vi "GenerateCode.vi"(1 "Terms":T1[](array[typedef]), 3 "Diagram":refnum<vi>, 5 "XRef":refnum<vi>, 6 "State In":T4) -> (0 "Generated Code?":bool, 2 "State Out":T4, 4 "Reply":string[](array[string]))   [LabVIEW 2012, in "Unindex and Unbundle.xnode"]
doc: "This ability VI is called when it is time to define the execution behavior of your XNode via LabVIEW's scripting API. This VI is only called when you have previously informed LabVIEW that you need to script through a GenerateCode reply. Diagram is a reference to a diagram of a temporary VI. This diagram contains exactly one front panel terminal for each terminal of your XNode. Terms is an array of pairs of Term IDs and terminal references. LabVIEW will copy code scripted into this diagram into your XNode and connect everything to the correct terminals. The front panel terminals that are on this diagram are special in that they can only be on the top level diagram.\n \n Generate Code? is used to tell LabVIEW whether or not you want to copy the scripted diagram over. If there is an error and you wish not to commit the changes, then the old XNode behavior will be left unchanged. If you set Generate Code? to false, then this VI will be called again next time type propagation is run. Otherwise, it will not be called until you indicate that it should be through the reply on another ability VI.\n \n Because the diagram you are scripting into is separate from the VI containing the XNode instance, type propagation and the data manager will run on the temporary VI after each scripting call.\n \n You should not use the Copy scripting method to move code into the temporary VI. This will adversely affect the user's clipboard. You should use the Move scripting method instead.\n\nDefault behavior: None.\n\nThis ability does not provide UI and OS messages are not handled.\n\nSee also: ModifyCode"
uses:
  Unindex and Unbundle.xnode
  State.ctl
  <vilib>/XNodeSupport/XNodeTermIDPair.ctl
  <vilib>/XNodeSupport/XNodeTermRef.ctl
  <vilib>/XNodeSupport/XNodeString.ctl
  <vilib>/Utility/miscctls.llb/LVPositionTypeDef.ctl
  VI Scripting/Scripting Tools/Scripting Tools.lvlib
  <vilib>/XNodeSupport/NI_XNodeSupport.lvlib
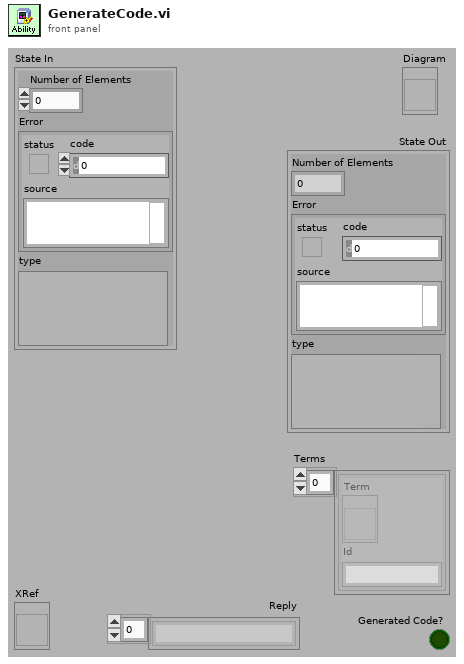
[diagram p1: front panel]
types:
  T1 = typedef "NI_XNodeSupport.lvlib/XNodeTermIDPair.ctl" = cluster{"Term":T2, "Id":T3}
  T2 = typedef "NI_XNodeSupport.lvlib/XNodeTermRef.ctl" = refnum<vi>
  T3 = typedef "NI_XNodeSupport.lvlib/XNodeString.ctl" = string
  T4 = typedef "Unindex and Unbundle.xnode/State.ctl" = cluster{"Number of Elements":i32, "Error":errorcluster, "type":variant}
  T5 = typedef "LVPositionTypeDef.ctl" = cluster{"Left":i32, "Top":i32}
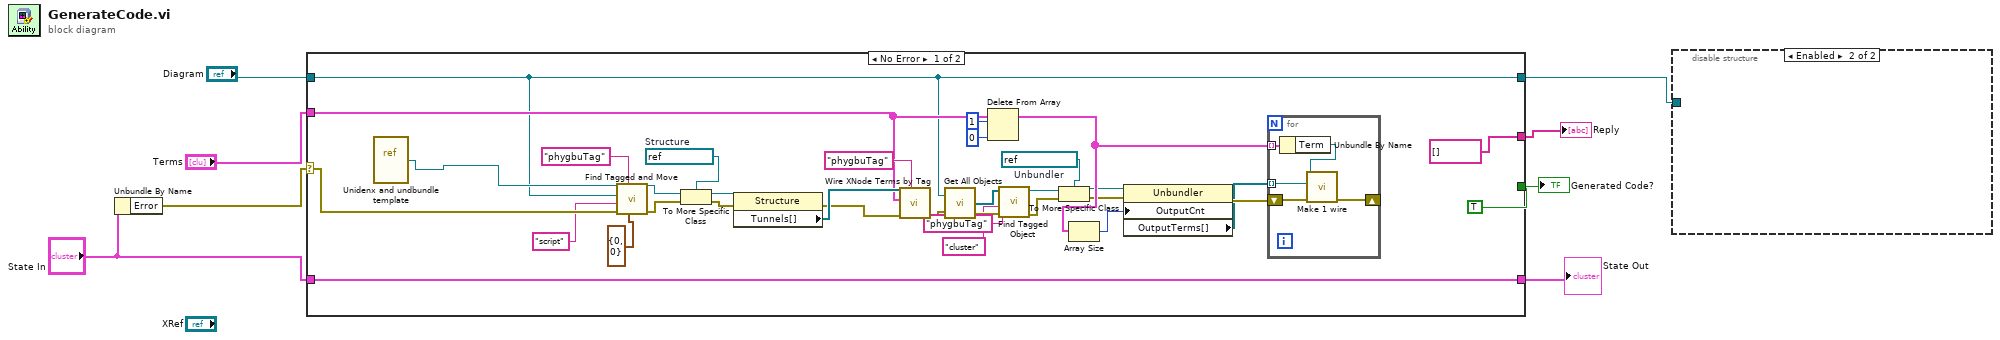
[diagram p0: block diagram]
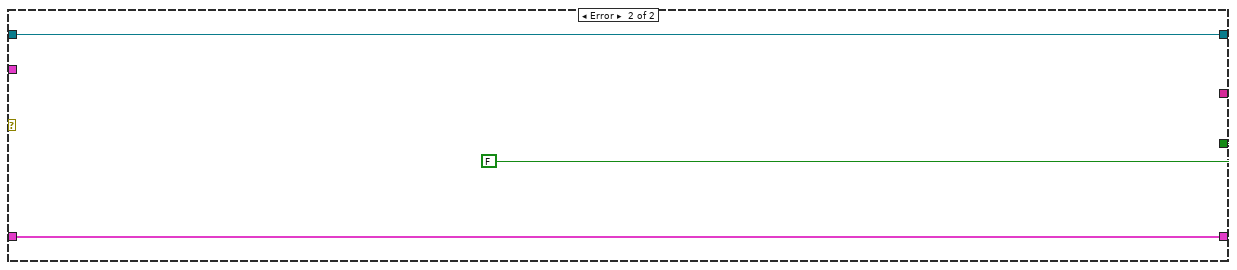
[diagram p2: hidden frame]
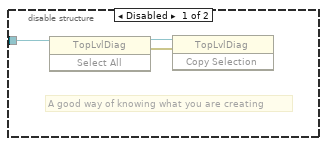
[diagram p3: hidden frame]
diagram:
  n1 = Unbundle By Name("State In") -> ("Error"=w1:errorcluster)
  n2 = case shown="No Error" w1 {
    selector: w1 -> [w36 _]
    tunnel: "State In" -> [w40 w50]
    tunnel: "Diagram" -> [w21 w48]
    tunnel: "Terms" -> [w26 _]
    tunnel: [w21 w48] -> w6
    tunnel: [string[] [] ("Reply") _] -> w5
    tunnel: [TRUE FALSE] -> w4
    tunnel: [w40 w50] -> w3
    frame No Error {
      w14 = refnum<vi> refnum  # Unbundler
      w38 = refnum<vi> refnum  # Structure
      n3 = vi-ref "Unidenx and undbundle template.vi"() -> (w27:refnum<vi>)
      n4 = call "Find Tagged and Move.vi"("position"=T5 {"Left"=0, "Top"=0}, "TagName"="phygbuTag", "error in"=w36, "TagValue"="script", "Destination Diagram"=w21, "VI Refnum"=w27) -> ("error out"=w31:errorcluster, "Moved Tagged object"=w32:refnum<vi>)  [unwired: 4 out]
      n5 = To More Specific Class(target class=w38, reference=w32, error in=w31) -> (specific class reference=w39:refnum<vi>, error out=w30:errorcluster)
      n6 = property class="Structure"(reference=w39, error in=w30) -> (error out=w29:errorcluster, "Tunnels[]"=w37:refnum<vi>[])  [unwired: 1 out]
      n7 = call "Wire XNode Terms by Tag.vi"("TagName"="phygbuTag", "error in (no error)"=w29, "Term Refs"=w26, "Source References"=w37) -> ("error out"=w23:errorcluster)  [unwired: 7 out]
      n8 = call "Get All Objects.vi"("Diagram In"=w21, "error in"=w23) -> ("All Objects"=w20:refnum<vi>[], "error out"=w22:errorcluster)  [unwired: 1 out]
      n9 = Delete From Array(array=w26, length=1, index=0) -> (array with subset deleted=w15:T1[])  [unwired: 1 out]
      n10 = call "Find Tagged Object.vi"("error in (no error)"=w22, "TagValue"="cluster", "TagName"="phygbuTag", "Array of References"=w20) -> ("error out"=w16:errorcluster, "reference"=w17:refnum<vi>)  [unwired: 1 in, 5 out]
      n11 = To More Specific Class(target class=w14, reference=w17, error in=w16) -> (specific class reference=w12:refnum<vi>, error out=w13:errorcluster)
      n12 = Array Size(array=w15) -> (size(s)=w10:i32)
      n13 = property class="Unbundler"(reference=w12, error in=w13, "OutputCnt"=w10) -> (error out=w11:errorcluster, "OutputTerms[]"=w9:refnum<vi>[])  [unwired: 1 out]
      n14 = for {
        shift-right: [w46] -> _
        shift-left: w11 -> [w47]
        tunnel: w15 -> [w45] mode=indexing
        tunnel: w9 -> [w43] mode=indexing
        n15 = Unbundle By Name(w45) -> ("Term"=w44:T2)
        n16 = call "Make 1 wire.vi"("error in"=w47, "Wire Terminal 2"=w43, "Wire Terminal 1"=w44) -> ("error out"=w46:errorcluster)  [unwired: 8 out]
      }
    }
    frame Error {
    }
  }
  "State Out" <- w3
  "Reply" <- w5
  "Generated Code?" <- w4
  n17 = disable-structure shown="Enabled" {
    disable-tunnel: w6 -> [w52 _]
    frame Disabled {
      # "A good way of knowing what you are creating"
      n18 = invoke class="TopLvlDiag" method="Select All"(reference=w52) -> (reference out=w53:refnum<vi>, error out=w51:errorcluster)  [unwired: 2 in, 1 out]
      n19 = invoke class="TopLvlDiag" method="Copy Selection"(reference=w53, error in=w51) -> ()  [unwired: 1 in, 3 out]
    }
    frame Enabled {
    }
  }
